vi "Archery_Game.vi"() -> ()   [LabVIEW 2014]
uses:
  <vilib>/Utility/cursorutil.llb/Set Cursor (Cursor ID).vi
  <vilib>/Utility/file.llb/Read From Spreadsheet File (string).vi
  <vilib>/Utility/file.llb/Write To Spreadsheet File (string).vi
panel:
  out "Arrow":bool
  out "radius":dbl
  out "theta":dbl
  in  "stop":bool
  out "MoveDir":bool
  out "Status":string
  out "Score":dbl
  out "PicT":i32
  out "PicL":i32
  out "BBound":dbl
  out "TBound":dbl=50.0
  out "RBound":dbl
  out "LBound":dbl=200.0
  out "ArrowDis":dbl
  out "Round":i32
  in  "Motion":T1(ring)
  out "MousePressed":bool
  out "Wind Intensity":dbl(slide) scale=0.0..1.0
  out "Wind Direction":dbl(knob)
  out "ScaleFactor":dbl=0.3
  out "picture show":picture caption="new picture"
  out "Intensity":dbl
  out "Direction":dbl
  out "Distance(m)":dbl
  out "Vertical":i32
  out "Horizontal":i32
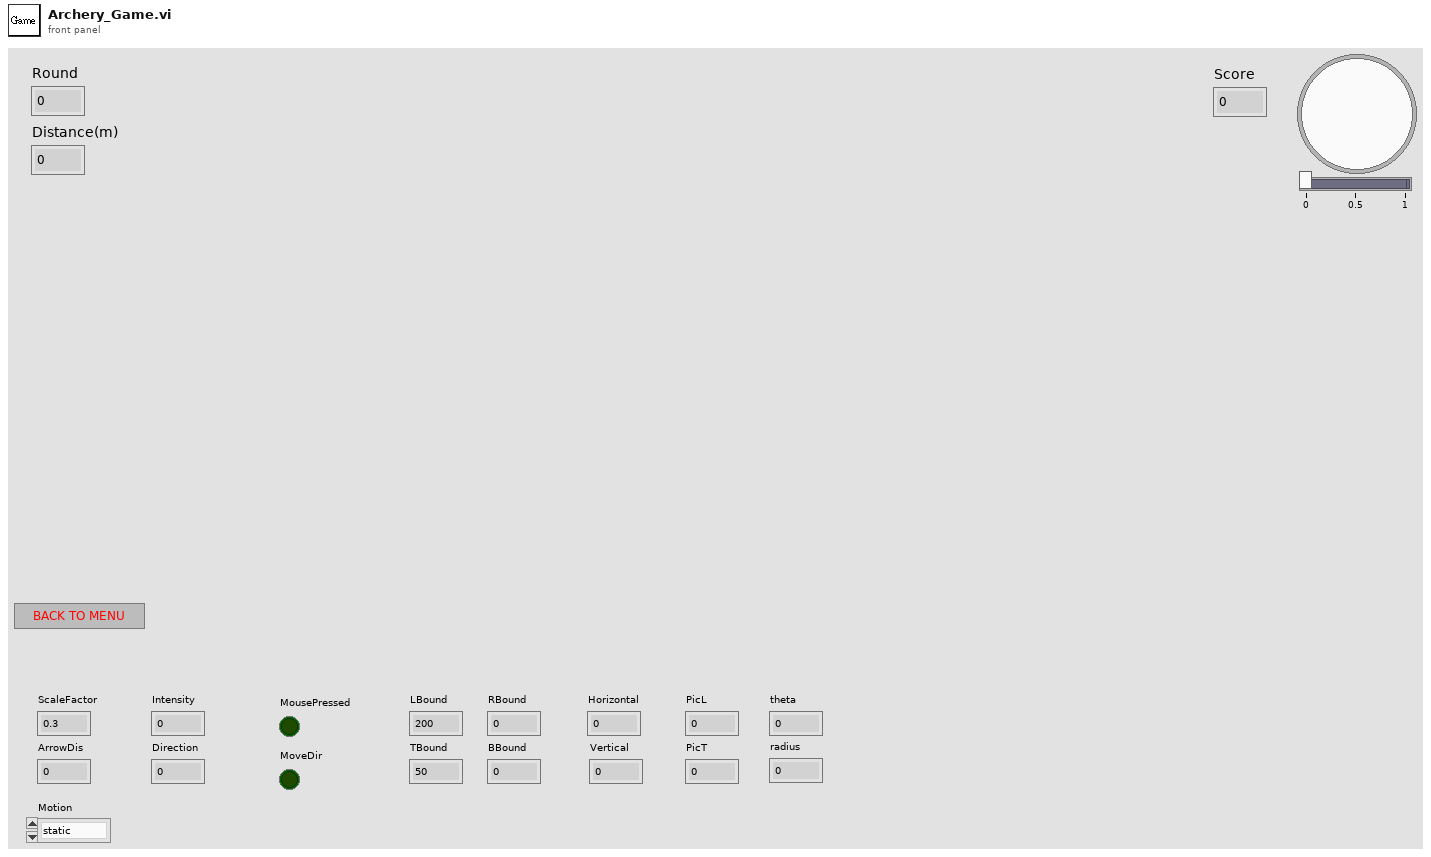
[diagram p1: front panel]
types:
  T1 = enum16{"static", "horizontal", "vertical", "circle"}
  T2 = typedef "imagedata.ctl" = cluster{"image type":i32, "image depth":i32, "image":u8[], "mask":u8[], "colors":u32[], "Rectangle":cluster{"left":i16, "top":i16, "right":i16, "bottom":i16}}
  T3 = typedef "LVPoint32TypeDef.ctl" = cluster{"Horizontal":i32, "Vertical":i32}
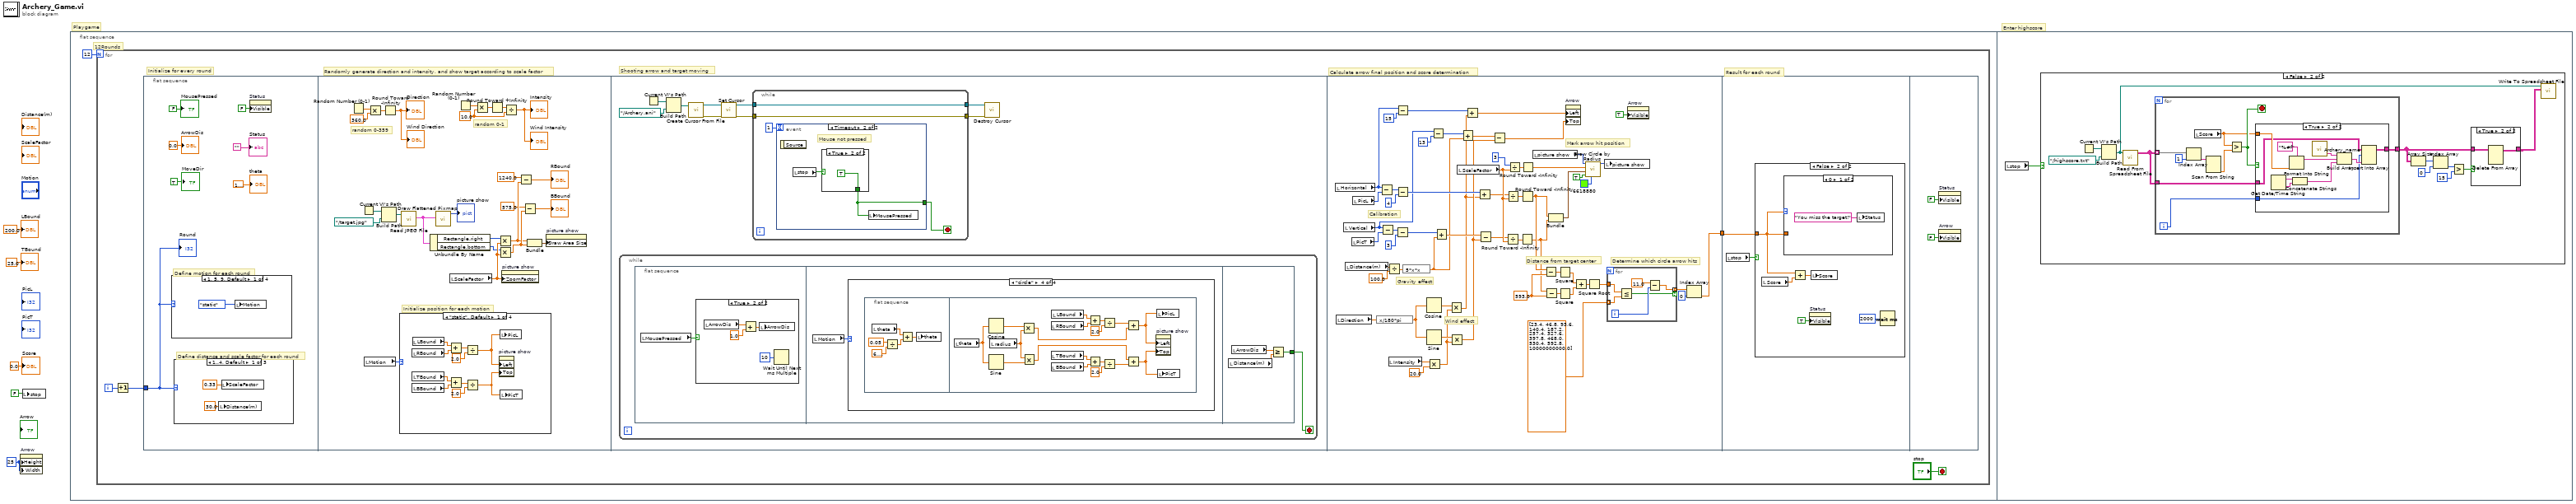
[diagram p0: block diagram]
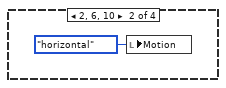
[diagram p2: hidden frame]
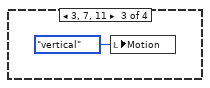
[diagram p3: hidden frame]
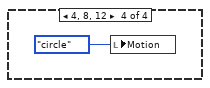
[diagram p4: hidden frame]
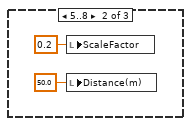
[diagram p5: hidden frame]
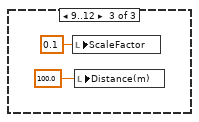
[diagram p6: hidden frame]
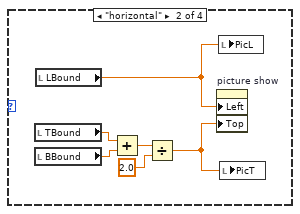
[diagram p7: hidden frame]
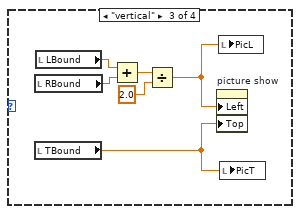
[diagram p8: hidden frame]
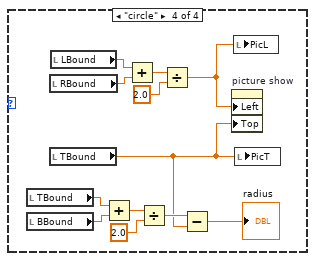
[diagram p9: hidden frame]
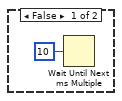
[diagram p10: hidden frame]
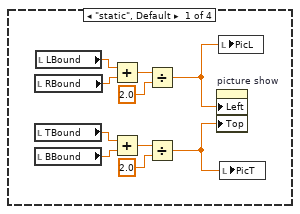
[diagram p11: hidden frame]
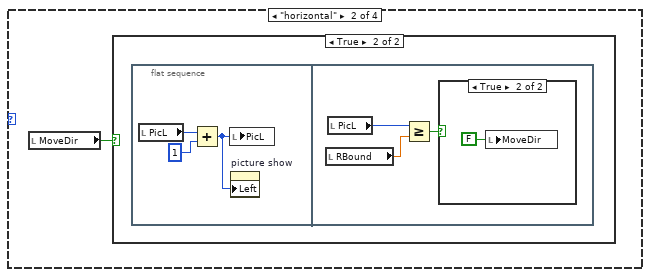
[diagram p12: hidden frame]
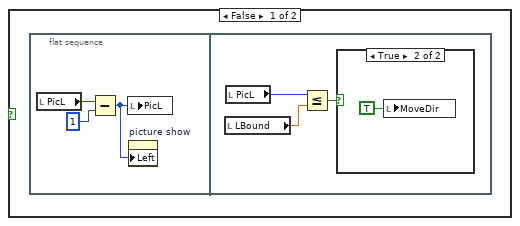
[diagram p13: hidden frame]
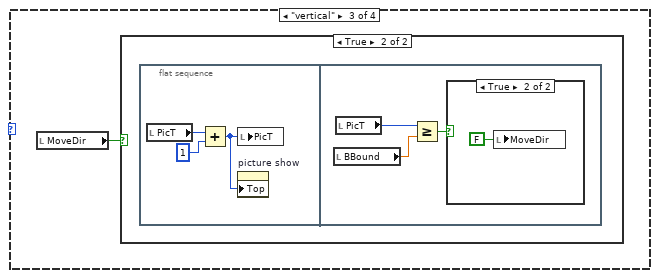
[diagram p16: hidden frame]
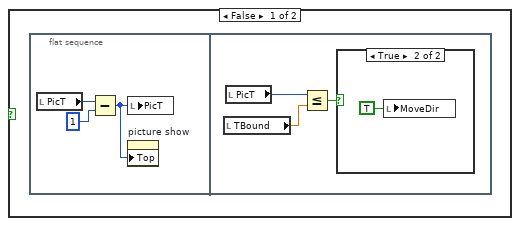
[diagram p17: hidden frame]
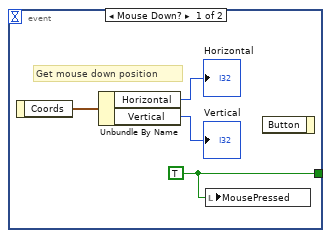
[diagram p20: hidden frame]
diagram:
  w1 = u32 25 ("Button Size:Height")
  # "Playgame"
  # "Enter highscore"
  n1 = property on="Arrow" class="Bool (strict)"("Height"=w1, "Width"=w1) -> ()  [unwired: 2 in, 2 out]
  n2 = local write "stop"(FALSE ("stop")) -> ()
  n3 = flat-sequence {
    frame #0 {
      # "12Rounds"
      n4 = for {
        N: 12 -> [_]
        i -> [w9]
        stop <- "stop" stop-if-true
        # "Result for each round"
        # "Calculate arrow final position and score determination"
        # "Initialize for every round"
        # "Randomly generate direction and intensity, and show target according to scale factor"
        # "Shooting arrow and target moving"
        n5 = Increment(x=w9) -> (x+1=w10:i32)
        n6 = flat-sequence {
          tunnel: w10 -> [w12]
          tunnel: [w197] -> w8
          tunnel: w8 -> [w247]
          frame #0 {
            # "Define distance and scale factor for each round"
            # "Define motion for each round"
            n7 = case shown="1, 5, 9, Default" w12 {
              frame 1, 5, 9, Default {
                n8 = local write "Motion"(T1."static") -> ()
              }
              frame 2, 6, 10 {
                n9 = local write "Motion"(T1."horizontal") -> ()
              }
              frame 3, 7, 11 {
                n10 = local write "Motion"(T1."vertical") -> ()
              }
              frame 4, 8, 12 {
                n11 = local write "Motion"(T1."circle") -> ()
              }
            }
            n12 = case shown="1..4, Default" w12 {
              frame 1..4, Default {
                n13 = local write "Distance(m)"(30.0 ("Distance")) -> ()
                n14 = local write "ScaleFactor"(0.33 ("ScaleFactor")) -> ()
              }
              frame 5..8 {
                n15 = local write "ScaleFactor"(0.2 ("ScaleFactor")) -> ()
                n16 = local write "Distance(m)"(50.0 ("Distance")) -> ()
              }
              frame 9..12 {
                n17 = local write "ScaleFactor"(0.1 ("ScaleFactor")) -> ()
                n18 = local write "Distance(m)"(100.0 ("Distance")) -> ()
              }
            }
            n19 = property on="Status" class="Str"("Visible"=FALSE) -> ()  [unwired: 2 in, 2 out]
            "MousePressed" <- FALSE ("BtnPressed")
            "ArrowDis" <- 0.0 ("ArrowDis")
            "MoveDir" <- TRUE ("MoveDir")
            "Status" <- ""
            "Round" <- w12
            "theta" <- 1.5707963267948966
          }
          frame #1 {
            w49 = 10.0 ("y")
            # "Initialize position for each motion"
            # "random 0-359"
            # "random 0-1"
            n20 = Random Number (0-1)() -> (number: 0 to 1=w46:dbl)
            n21 = Current VI's Path() -> (path=w30:path)
            n22 = local read "Motion"() -> (w28:T1)
            n23 = Multiply(x=w46, y=360.0) -> (x*y=w47:dbl)
            n24 = Build Path(base path=w30, name or relative path=path "../target.jpg") -> (appended path=w31:path)
            n25 = Round Toward -Infinity(1:w47) -> (0:→"Wind Direction" →"Direction":dbl)
            n26 = case shown="\"static\", Default" w28 {
              frame "static", Default {
                n27 = local read "RBound"() -> (w61:dbl)
                n28 = local read "TBound"() -> (w55:dbl)
                n29 = local read "BBound"() -> (w56:dbl)
                n30 = local read "LBound"() -> (w62:dbl)
                n31 = Add(x=w62, y=w61) -> (x+y=w60:dbl)
                n32 = Add(x=w55, y=w56) -> (x+y=w57:dbl)
                n33 = Divide(x=w60, y=2.0) -> (x/y=w54:dbl)
                n34 = Divide(x=w57, y=2.0) -> (x/y=w53:dbl)
                n35 = property on="picture show" class="Pict"("Left"=w54, "Top"=w53) -> ()  [unwired: 2 in, 2 out]
                n36 = local write "PicL"(w54) -> ()
                n37 = local write "PicT"(w53) -> ()
              }
              frame "horizontal" {
                n38 = local read "TBound"() -> (w65:dbl)
                n39 = local read "BBound"() -> (w66:dbl)
                n40 = local read "LBound"() -> (w63:dbl)
                n41 = Add(x=w65, y=w66) -> (x+y=w67:dbl)
                n42 = Divide(x=w67, y=2.0) -> (x/y=w64:dbl)
                n43 = property on="picture show" class="Pict"("Left"=w63, "Top"=w64) -> ()  [unwired: 2 in, 2 out]
                n44 = local write "PicL"(w63) -> ()
                n45 = local write "PicT"(w64) -> ()
              }
              frame "vertical" {
                n46 = local read "RBound"() -> (w73:dbl)
                n47 = local read "TBound"() -> (w69:dbl)
                n48 = local read "LBound"() -> (w74:dbl)
                n49 = Add(x=w74, y=w73) -> (x+y=w72:dbl)
                n50 = Divide(x=w72, y=2.0) -> (x/y=w70:dbl)
                n51 = property on="picture show" class="Pict"("Left"=w70, "Top"=w69) -> ()  [unwired: 2 in, 2 out]
                n52 = local write "PicL"(w70) -> ()
                n53 = local write "PicT"(w69) -> ()
              }
              frame "circle" {
                n54 = local read "TBound"() -> (w78:dbl)
                n55 = local read "BBound"() -> (w79:dbl)
                n56 = local read "RBound"() -> (w85:dbl)
                n57 = local read "TBound"() -> (w75:dbl)
                n58 = local read "LBound"() -> (w86:dbl)
                n59 = Add(x=w78, y=w79) -> (x+y=w80:dbl)
                n60 = Add(x=w86, y=w85) -> (x+y=w84:dbl)
                n61 = Divide(x=w80, y=2.0) -> (x/y=w76:dbl)
                n62 = Divide(x=w84, y=2.0) -> (x/y=w82:dbl)
                n63 = Subtract(x=w76, y=w75) -> (x-y=→"radius":dbl)
                n64 = property on="picture show" class="Pict"("Left"=w82, "Top"=w75) -> ()  [unwired: 2 in, 2 out]
                n65 = local write "PicL"(w82) -> ()
                n66 = local write "PicT"(w75) -> ()
              }
            }
            n67 = call <vilib>:"Read JPEG File.vi"("path to JPEG file"=w31) -> ("image data"=w29:T2)  [unwired: 8 in, 2 out]
            n68 = Unbundle By Name(w29) -> ("Rectangle.right"=w42:i16, "Rectangle.bottom"=w43:i16)
            n69 = call <vilib>:"Draw Flattened Pixmap.vi"("image data"=w29) -> ("new picture"=→"picture show":picture)  [unwired: 8 in]
            n70 = local read "ScaleFactor"() -> (w44:dbl)
            n71 = Random Number (0-1)() -> (number: 0 to 1=w52:dbl)
            n72 = Multiply(x=w52, y=w49) -> (x*y=w51:dbl)
            n73 = Round Toward +Infinity(x=w51) -> (ceil(x): smallest int >= x=w50:dbl)
            n74 = Multiply(x=w42, y=w44) -> (x*y=w37:dbl)
            n75 = Multiply(x=w43, y=w44) -> (x*y=w38:dbl)
            n76 = property on="picture show" class="Pict"("ZoomFactor"=w44) -> ()  [unwired: 2 in, 2 out]
            n77 = Divide(x=w50, y=w49) -> (x/y=→"Wind Intensity" →"Intensity":dbl)
            n78 = Subtract(x=1240.0, y=w37) -> (x-y=→"RBound":dbl)
            n79 = Subtract(x=575.0, y=w38) -> (x-y=→"BBound":dbl)
            n80 = Bundle(w37, w38) -> (w41:cluster{dbl, dbl})  [unwired: 1 in]
            n81 = property on="picture show" class="Pict"("Draw Area Size"=w41) -> ()  [unwired: 2 in, 2 out]
          }
          frame #2 {
            n82 = while {
              stop <- w96 stop-if-true
              n83 = flat-sequence {
                tunnel: [w167] -> w96
                frame #0 {
                  n84 = local read "MousePressed"() -> (w97:bool)
                  n85 = case shown="True" w97 {
                    frame False {
                      n86 = Wait Until Next ms Multiple(millisecond multiple=u32 10) -> ()  [unwired: 1 out]
                    }
                    frame True {
                      n87 = local read "ArrowDis"() -> (w102:dbl)
                      n88 = Add(x=w102, y=1.0) -> (x+y=w101:dbl)
                      n89 = local write "ArrowDis"(w101) -> ()
                      n90 = Wait Until Next ms Multiple(millisecond multiple=u32 10) -> ()  [unwired: 1 out]
                    }
                  }
                }
                frame #1 {
                  n91 = local read "Motion"() -> (w103:T1)
                  n92 = case shown="\"circle\"" w103 {
                    frame "static", Default {
                      n93 = local read "RBound"() -> (w105:dbl)
                      n94 = local read "TBound"() -> (w111:dbl)
                      n95 = local read "BBound"() -> (w110:dbl)
                      n96 = local read "LBound"() -> (w104:dbl)
                      n97 = Add(x=w104, y=w105) -> (x+y=w106:dbl)
                      n98 = Add(x=w111, y=w110) -> (x+y=w109:dbl)
                      n99 = Divide(x=w106, y=2.0) -> (x/y=w112:dbl)
                      n100 = Divide(x=w109, y=2.0) -> (x/y=w113:dbl)
                      n101 = property on="picture show" class="Pict"("Left"=w112, "Top"=w113) -> ()  [unwired: 2 in, 2 out]
                      n102 = local write "PicL"(w112) -> ()
                      n103 = local write "PicT"(w113) -> ()
                    }
                    frame "horizontal" {
                      n104 = local read "MoveDir"() -> (w114:bool)
                      n105 = case shown="True" w114 {
                        frame False {
                          n106 = flat-sequence {
                            frame #0 {
                              n107 = local read "PicL"() -> (w116:i32)
                              n108 = Subtract(x=w116, y=1) -> (x-y=w115:i32)
                              n109 = local write "PicL"(w115) -> ()
                              n110 = property on="picture show" class="Pict"("Left"=w115) -> ()  [unwired: 2 in, 2 out]
                            }
                            frame #1 {
                              n111 = local read "LBound"() -> (w119:dbl)
                              n112 = local read "PicL"() -> (w120:i32)
                              n113 = Less Or Equal?(x=w120, y=w119) -> (x <= y?=w118:bool)
                              n114 = case shown="True" w118 {
                                frame False {
                                }
                                frame True {
                                n115 = local write "MoveDir"(TRUE ("MoveDir")) -> ()
                                }
                              }
                            }
                          }
                        }
                        frame True {
                          n116 = flat-sequence {
                            frame #0 {
                              n117 = local read "PicL"() -> (w123:i32)
                              n118 = Add(x=w123, y=1) -> (x+y=w122:i32)
                              n119 = local write "PicL"(w122) -> ()
                              n120 = property on="picture show" class="Pict"("Left"=w122) -> ()  [unwired: 2 in, 2 out]
                            }
                            frame #1 {
                              n121 = local read "RBound"() -> (w126:dbl)
                              n122 = local read "PicL"() -> (w127:i32)
                              n123 = Greater Or Equal?(x=w127, y=w126) -> (x >= y?=w125:bool)
                              n124 = case shown="True" w125 {
                                frame False {
                                }
                                frame True {
                                n125 = local write "MoveDir"(FALSE ("MoveDir")) -> ()
                                }
                              }
                            }
                          }
                        }
                      }
                    }
                    frame "vertical" {
                      n126 = local read "MoveDir"() -> (w129:bool)
                      n127 = case shown="True" w129 {
                        frame False {
                          n128 = flat-sequence {
                            frame #0 {
                              n129 = local read "PicT"() -> (w131:i32)
                              n130 = Subtract(x=w131, y=1) -> (x-y=w130:i32)
                              n131 = local write "PicT"(w130) -> ()
                              n132 = property on="picture show" class="Pict"("Top"=w130) -> ()  [unwired: 2 in, 2 out]
                            }
                            frame #1 {
                              n133 = local read "TBound"() -> (w134:dbl)
                              n134 = local read "PicT"() -> (w135:i32)
                              n135 = Less Or Equal?(x=w135, y=w134) -> (x <= y?=w133:bool)
                              n136 = case shown="True" w133 {
                                frame False {
                                }
                                frame True {
                                n137 = local write "MoveDir"(TRUE ("MoveDir")) -> ()
                                }
                              }
                            }
                          }
                        }
                        frame True {
                          n138 = flat-sequence {
                            frame #0 {
                              n139 = local read "PicT"() -> (w138:i32)
                              n140 = Add(x=w138, y=1) -> (x+y=w137:i32)
                              n141 = local write "PicT"(w137) -> ()
                              n142 = property on="picture show" class="Pict"("Top"=w137) -> ()  [unwired: 2 in, 2 out]
                            }
                            frame #1 {
                              n143 = local read "BBound"() -> (w141:dbl)
                              n144 = local read "PicT"() -> (w142:i32)
                              n145 = Greater Or Equal?(x=w142, y=w141) -> (x >= y?=w140:bool)
                              n146 = case shown="True" w140 {
                                frame False {
                                }
                                frame True {
                                n147 = local write "MoveDir"(FALSE ("MoveDir")) -> ()
                                }
                              }
                            }
                          }
                        }
                      }
                    }
                    frame "circle" {
                      n148 = flat-sequence {
                        frame #0 {
                          n149 = local read "theta"() -> (w148:dbl)
                          n150 = Divide(x=0.05, y=6.283185307179586) -> (x/y=w146:dbl)
                          n151 = Add(x=w148, y=w146) -> (x+y=w147:dbl)
                          n152 = local write "theta"(w147) -> ()
                        }
                        frame #1 {
                          n153 = local read "theta"() -> (w166:dbl)
                          n154 = Sine(x=w166) -> (sin(x)=w165:dbl)
                          n155 = Cosine(x=w166) -> (cos(x)=w164:dbl)
                          n156 = local read "radius"() -> (w163:dbl)
                          n157 = Multiply(x=w164, y=w163) -> (x*y=w151:dbl)
                          n158 = Multiply(x=w163, y=w165) -> (x*y=w153:dbl)
                          n159 = local read "RBound"() -> (w156:dbl)
                          n160 = local read "TBound"() -> (w162:dbl)
                          n161 = local read "BBound"() -> (w161:dbl)
                          n162 = local read "LBound"() -> (w155:dbl)
                          n163 = Add(x=w155, y=w156) -> (x+y=w157:dbl)
                          n164 = Add(x=w162, y=w161) -> (x+y=w160:dbl)
                          n165 = Divide(x=w157, y=2.0) -> (x/y=w152:dbl)
                          n166 = Divide(x=w160, y=2.0) -> (x/y=w154:dbl)
                          n167 = Add(x=w152, y=w151) -> (x+y=w150:dbl)
                          n168 = Add(x=w153, y=w154) -> (x+y=w149:dbl)
                          n169 = property on="picture show" class="Pict"("Left"=w150, "Top"=w149) -> ()  [unwired: 2 in, 2 out]
                          n170 = local write "PicL"(w150) -> ()
                          n171 = local write "PicT"(w149) -> ()
                        }
                      }
                    }
                  }
                }
                frame #2 {
                  n172 = local read "Distance(m)"() -> (w169:dbl)
                  n173 = local read "ArrowDis"() -> (w168:dbl)
                  n174 = Greater Or Equal?(x=w168, y=w169) -> (x >= y?=w167:bool)
                }
              }
            }
            n175 = Current VI's Path() -> (path=w89:path)
            n176 = Build Path(base path=w89, name or relative path=path "../Archery.ani") -> (appended path=w87:path)
            n177 = call <vilib>:"Create Cursor From File.vi"("cursor file"=w87) -> ("error out"=w90:errorcluster, "cursor ID"=w91:refnum<k1>)  [unwired: 9 in]
            n178 = call-poly <vilib>:"Set Cursor.vi"("error in (no error)"=w90, "cursor ID"=w91) -> ("error out"=w93:errorcluster, "previous cursor ID"=w95:refnum<k1>)  [unwired: 8 in]
            n179 = while {
              tunnel: [w173] -> w94
              tunnel: w95 -> [w173]
              tunnel: [w172] -> w92
              tunnel: w93 -> [w172]
              stop <- w170 stop-if-true
              n180 = event shown="[1] Timeout" {
                selector: _ -> [_ _]
                dyn-events: _ -> [_ _]
                timeout: 1 -> [_ _]
                tunnel: [w174 w178] -> w170
                event Mouse Down? {
                  w174 = TRUE
                  # "Get mouse down position"
                  n181 = event-data() -> ("Coords"=w177:T3)  [unwired: 1 in]
                  n182 = Unbundle By Name(w177) -> ("Horizontal"=→"Horizontal":i32, "Vertical"=→"Vertical":i32)
                  n183 = local write "MousePressed"(w174) -> ()
                  n184 = event-data() -> ()  [unwired: 2 in, 1 out]
                }
                event Timeout {
                  # "Mouse not pressed"
                  n185 = event-data() -> ()  [unwired: 1 in, 1 out]
                  n186 = local read "stop"() -> (w179:bool)
                  n187 = case shown="True" w179 {
                    tunnel: [FALSE TRUE] -> w178
                    frame False {
                    }
                    frame True {
                    }
                  }
                  n188 = local write "MousePressed"(w178) -> ()
                }
              }
            }
            n189 = call <vilib>:"Destroy Cursor.vi"("cursor ID"=w94, "error in (no error)"=w92) -> ()  [unwired: 8 in, 1 out]
          }
          frame #3 {
            w211 = 593.0 ("y")
            # "Mark arrow hit position"
            # "Determine which circle arrow hits"
            # "Distance from target center"
            # "Wind effect"
            # "Gravity effect"
            # "Calibration"
            n190 = local read "Horizontal"() -> (w194:i32)
            n191 = local read "Direction"() -> (w219:dbl)
            n192 = local read "Vertical"() -> (w192:i32)
            n193 = local read "Distance(m)"() -> (w223:dbl)
            n194 = local read "PicT"() -> (w235:i32)
            n195 = local read "PicL"() -> (w236:i32)
            n196 = expression code="x/180*pi"(w219) -> (w212:dbl)
            n197 = Subtract(x=w194, y=w236) -> (x-y=w231:i32)
            n198 = Subtract(x=w192, y=w235) -> (x-y=w230:i32)
            n199 = Divide(x=w223, y=100.0) -> (x/y=w221:dbl)
            n200 = local read "Intensity"() -> (w218:dbl)
            n201 = Subtract(x=w230, y=3) -> (x-y=w209:i32)
            n202 = Subtract(x=w194, y=15) -> (x-y=w185:i32)
            n203 = Subtract(x=w231, y=4) -> (x-y=w210:i32)
            n204 = expression code="5*x*x"(w221) -> (w190:dbl)
            n205 = Cosine(x=w212) -> (cos(x)=w215:dbl)
            n206 = Sine(x=w212) -> (sin(x)=w216:dbl)
            n207 = Multiply(x=w218, y=20.0) -> (x*y=w214:dbl)
            n208 = Subtract(x=w192, y=13) -> (x-y=w189:i32)
            n209 = Add(x=w209, y=w190) -> (x+y=w213:dbl)
            n210 = Multiply(x=w215, y=w214) -> (x*y=w186:dbl)
            n211 = Multiply(x=w216, y=w214) -> (x*y=w188:dbl)
            n212 = local read "ScaleFactor"() -> (w225:dbl)
            n213 = Add(x=w189, y=w190) -> (x+y=w187:dbl)
            n214 = Add(x=w185, y=w186) -> (x+y=w184:dbl)
            n215 = Add(x=w210, y=w186) -> (x+y=w195:dbl)
            n216 = Subtract(x=w213, y=w188) -> (x-y=w196:dbl)
            n217 = Subtract(x=w187, y=w188) -> (x-y=w183:dbl)
            n218 = Divide(x=w196, y=w225) -> (x/y=w232:dbl)
            n219 = Divide(x=w195, y=w225) -> (x/y=w233:dbl)
            n220 = Divide(x=i16 3 ("radius"), y=w225) -> (x/y=w226:dbl)
            n221 = Round Toward -Infinity(1:w232) -> (0:w198:dbl)
            n222 = Round Toward -Infinity(1:w233) -> (0:w199:dbl)
            n223 = Round Toward -Infinity(1:w226) -> (0:w224:dbl)
            n224 = local read "picture show"() -> (w239:picture)
            n225 = Subtract(x=w199, y=w211) -> (x-y=w208:dbl)
            n226 = Subtract(x=w198, y=w211) -> (x-y=w207:dbl)
            n227 = Bundle(w199, w198) -> (w220:cluster{dbl, dbl})  [unwired: 1 in]
            n228 = Square(x=w208) -> (x^2=w205:dbl)
            n229 = Square(x=w207) -> (x^2=w206:dbl)
            n230 = property on="Arrow" class="Bool (strict)"("Left"=w184, "Top"=w183) -> ()  [unwired: 2 in, 2 out]
            n231 = Add(x=w205, y=w206) -> (x+y=w204:dbl)
            n232 = call <vilib>:"Draw Circle by Radius.vi"("color(black)"=u32 6618880, "fill?(F)"=TRUE, "pixel center"=w220, "radius"=w224, "picture"=w239) -> ("new picture"=w238:picture)  [unwired: 6 in]
            n233 = Square Root(x=w204) -> (sqrt(x)=w200:dbl)
            n234 = local write "picture show"(w238) -> ()
            n235 = for {
              tunnel: dbl[] [23.4, 46.8, 93.6, 140.4, 187.2, 257.4, 327.6, 397.8, 468.0, 530.4, 592.8, 10000000000.0] -> [w241] mode=indexing
              tunnel: w200 -> [w242]
              tunnel: [w243] -> w202 mode=indexing if=w240
              i -> [w244]
              n236 = Less Or Equal?(x=w242, y=w241) -> (x <= y?=w240:bool)
              n237 = Subtract(x=11.0, y=w244) -> (x-y=w243:dbl)
            }
            n238 = property on="Arrow" class="Bool (strict)"("Visible"=TRUE) -> ()  [unwired: 2 in, 2 out]
            n239 = Index Array(array=w202, index=0) -> (element=w197:dbl)
          }
          frame #4 {
            n240 = local read "stop"() -> (w246:bool)
            n241 = case shown="False" w246 {
              tunnel: w247 -> [_ w250]
              frame True {
              }
              frame False {
                n242 = local read "Score"() -> (w252:dbl)
                n243 = case shown="0" w250 {
                  tunnel: w250 -> [_ w255]
                  frame 0 {
                    n244 = local write "Status"("You miss the target!" ("message")) -> ()
                  }
                  frame 1, Default {
                    n245 = Format Into String(format string="You get %#f points!", w255) -> (resulting string=w254:string)  [unwired: 2 in, 1 out]
                    n246 = local write "Status"(w254) -> ()
                  }
                }
                n247 = Add(x=w250, y=w252) -> (x+y=w251:dbl)
                n248 = property on="Status" class="Str"("Visible"=TRUE) -> ()  [unwired: 2 in, 2 out]
                n249 = local write "Score"(w251) -> ()
                n250 = Wait (ms)(milliseconds to wait=u32 2000) -> ()  [unwired: 1 out]
              }
            }
          }
          frame #5 {
            n251 = property on="Status" class="Str"("Visible"=FALSE) -> ()  [unwired: 2 in, 2 out]
            n252 = property on="Arrow" class="Bool (strict)"("Visible"=FALSE) -> ()  [unwired: 2 in, 2 out]
          }
        }
      }
    }
    frame #1 {
      n253 = local read "stop"() -> (w259:bool)
      n254 = case shown="False" w259 {
        frame True {
          # "Exit by user, so no need to record highscore"
        }
        frame False {
          n255 = Current VI's Path() -> (path=w270:path)
          n256 = Build Path(base path=w270, name or relative path=path "../highscore.txt") -> (appended path=w267:path)
          n257 = call-poly <vilib>:"Read From Spreadsheet File.vi"("file path (dialog if empty)"=w267) -> ("all rows"=w268:string[][])  [unwired: 6 in, 4 out]
          n258 = for {
            tunnel: w268 -> [w278] mode=indexing
            tunnel: w268 -> [w275]
            tunnel: [w274] -> w262
            i -> [w276]
            stop <- w279 stop-if-true
            n259 = Index Array(array=w278, index=1) -> (element=w281:string)
            n260 = local read "Score"() -> (w277:dbl)
            n261 = Scan From String(input string=w281) -> (output 1=w280:dbl)  [unwired: 4 in, 3 out]
            n262 = Greater?(x=w277, y=w280) -> (0:w279:bool)
            n263 = case shown="True" w279 {
              tunnel: w275 -> [w283 w288]
              tunnel: w277 -> [_ w294]
              tunnel: w276 -> [_ w287]
              tunnel: [w283 w286] -> w274
              frame False {
              }
              frame True {
                n264 = Get Date/Time String() -> (date string=w292:string, time string=w291:string)  [unwired: 3 in]
                n265 = Format Into String(format string="%#f", w294) -> (resulting string=w293:string)  [unwired: 2 in, 1 out]
                n266 = Concatenate Strings(w292, w291) -> (w290:string)
                n267 = call "Archery_name.vi"() -> ("Enter Name Ind"=w284:string)  [unwired: 3 in]
                n268 = Build Array(w284, w293, w290) -> (w289:string[])
                n269 = Insert Into Array(array=w288, index (row)=w287, new element=w289) -> (w286:string[][])  [unwired: 1 in]
              }
            }
          }
          n270 = Array Size(array=w262) -> (size(s)=w266:i32[])
          n271 = Index Array(array=w266, index=0) -> (element=w264:i32)
          n272 = Greater?(x=w264, y=15) -> (0:w260:bool)
          n273 = case shown="True" w260 {
            tunnel: w262 -> [w271 w273]
            tunnel: [w271 w272] -> w261
            frame False {
            }
            frame True {
              n274 = Delete From Array(array=w273) -> (array with subset deleted=w272:string[][])  [unwired: 3 in, 1 out]
            }
          }
          n275 = call-poly <vilib>:"Write To Spreadsheet File.vi"("2D data"=w261, "file path (dialog if empty)"=w267) -> ()  [unwired: 6 in, 1 out]
        }
      }
    }
  }
  "LBound" <- 200.0 ("LBound")
  "TBound" <- 25.0 ("TBound")
  "Score" <- 0.0 ("Score")
